vi "3D - C (SubVI).vi"(10 "Angle theta":dbl, 11 "Magnitude":dbl) -> (3 "B_C":dbl format="%#_6f")   [LabVIEW 2018]
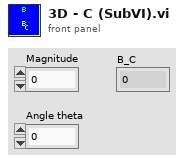
[diagram p1: front panel]
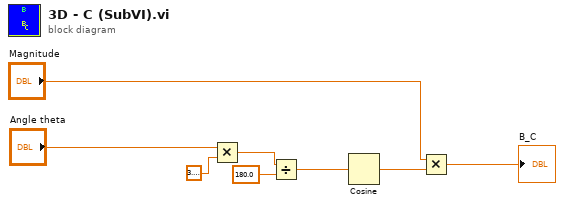
[diagram p0: block diagram]
diagram:
  n1 = Multiply(x="Angle theta", y=3.141592653589793) -> (x*y=w3:dbl)
  n2 = Divide(x=w3, y=180.0) -> (x/y=w5:dbl)
  n3 = Cosine(x=w5) -> (cos(x)=w6:dbl)
  n4 = Multiply(x="Magnitude", y=w6) -> (x*y=→"B_C":dbl)
